vi "CalculateDiscount.vi"(8 "Error In":errorcluster, 9 "CurrentDiscount":ext, 10 "Customer":refnum<class "Customer.lvclass">, 11 "object in":refnum<class "IDiscountRule.lvclass">) -> (0 "Error Out":errorcluster, 2 "Return(EXT)":ext, 3 "object out":refnum<class "IDiscountRule.lvclass">)   [LabVIEW 2020, in "IDiscountRule.lvclass"]
uses:
  IDiscountRule.lvclass
  Customer_class/Customer.lvclass
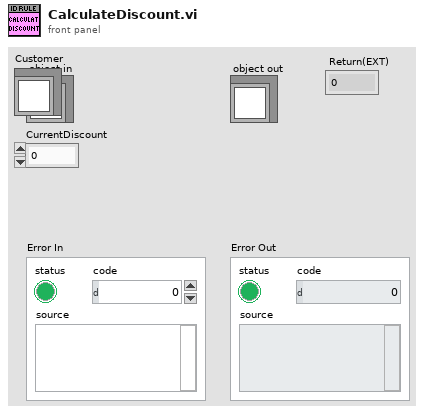
[diagram p1: front panel]
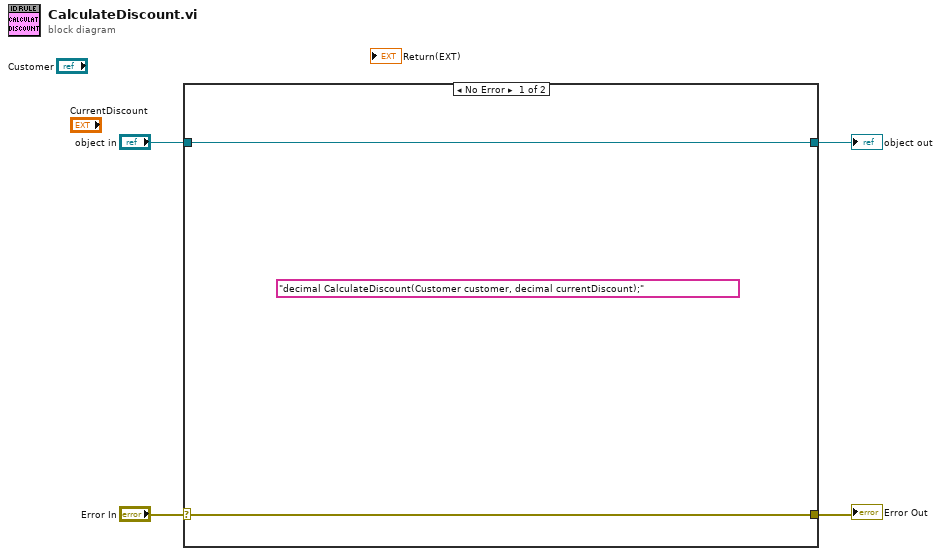
[diagram p0: block diagram]
diagram:
  (unwired) "decimal CalculateDiscount(Customer customer, decimal currentDiscount);"
  n1 = case shown="No Error" "Error In" {
    selector: "Error In" -> [w6 w8]
    tunnel: [w6 w8] -> w3
    tunnel: [w5 w7] -> w1
    tunnel: "object in" -> [w5 w7]
    frame No Error {
    }
    frame Error {
    }
  }
  "Error Out" <- w3
  "object out" <- w1
